vi "html_read.vi"() -> ()   [LabVIEW 2015]
uses:
  <vilib>/httpClient/LabVIEWHTTPClient.lvlib
panel:
  out "body 2":string
  in  "File Type":string=".CSV"
  in  "File Prefix":string="GPSLOG"
  out "Number of Files":i32
  out "body":string
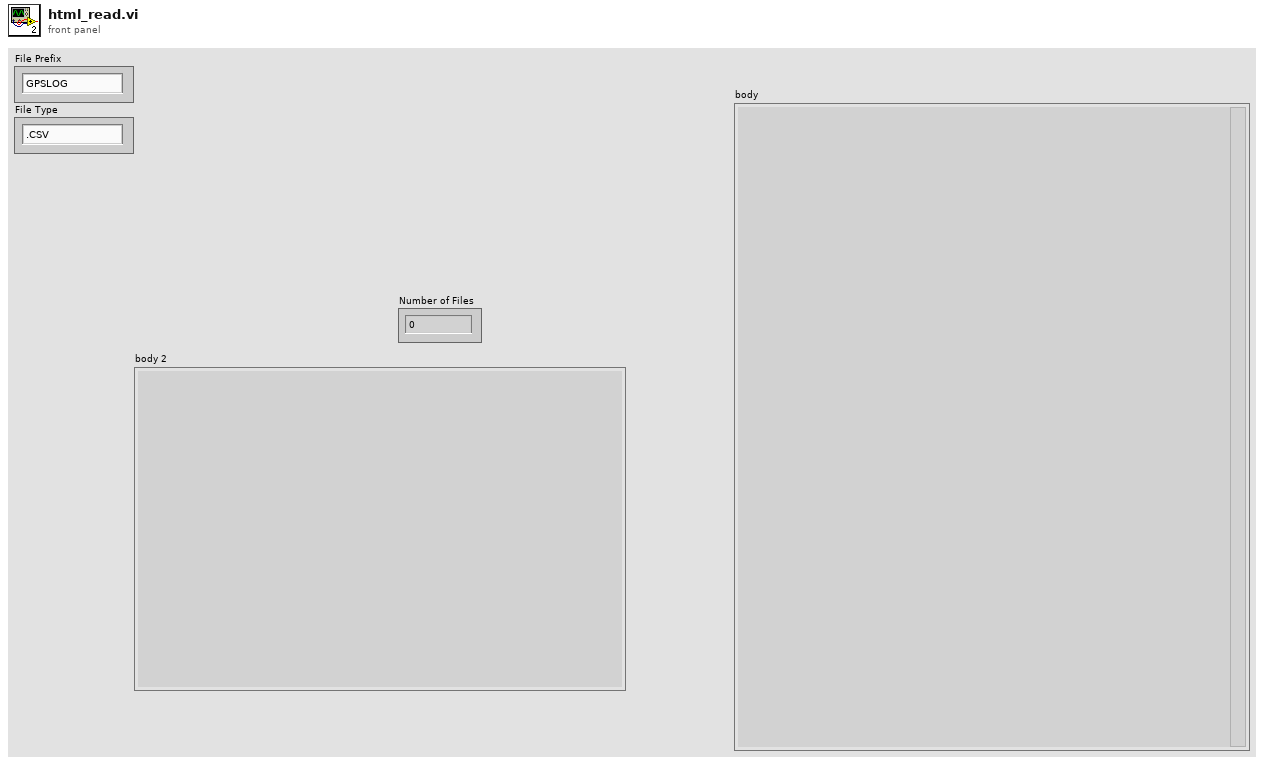
[diagram p1: front panel]
types:
  T1 = typedef "LabVIEWHTTPClient.lvlib/ClientHandle.ctl" = refnum<k1>
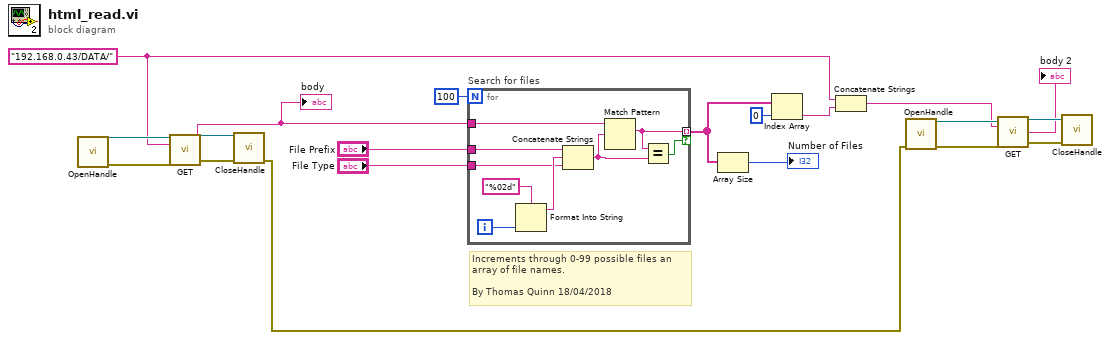
[diagram p0: block diagram]
diagram:
  w4 = "192.168.0.43/DATA/" ("url")
  # "Increments through 0-99 possible files an array of file names.\n\nBy Thomas Quinn 18/04/2018"
  n1 = call <vilib>:"OpenHandle.vi"() -> ("client handle out"=w20:T1, "error out"=w19:errorcluster)  [unwired: 14 in]
  n2 = call <vilib>:"GET.vi"("client handle"=w20, "url"=w4, "error in (no error)"=w19) -> ("client handle out"=w13:T1, "body"=w17:string, "error out"=w12:errorcluster)  [unwired: 9 in, 1 out]
  "body" <- w17
  n3 = call <vilib>:"CloseHandle.vi"("client handle"=w13, "error in (no error)"=w12) -> ("error out"=w9:errorcluster)  [unwired: 13 in]
  n4 = for "Search for files" {
    N: 100 -> [_]
    tunnel: "File Prefix" -> [w26]
    tunnel: w17 -> [w29]
    tunnel: [w21] -> w6 mode=indexing if=w22
    tunnel: "File Type" -> [w24]
    i -> [w28]
    n5 = Format Into String(format string="%02d", w28) -> (resulting string=w25:string)  [unwired: 2 in, 1 out]
    n6 = Concatenate Strings(w26, w25, w24) -> (w23:string)
    n7 = Match Pattern(string=w29, regular expression=w23) -> (match substring=w21:string)  [unwired: 1 in, 3 out]
    n8 = Equal?(x=w21, y=w23) -> (x = y?=w22:bool)
  }
  n9 = Array Size(array=w6) -> (size(s)=→"Number of Files":i32)
  n10 = Index Array(array=w6, index=0) -> (element=w3:string)
  n11 = Concatenate Strings(w4, w3) -> (w2:string)
  n12 = call <vilib>:"OpenHandle.vi"("error in (no error)"=w9) -> ("client handle out"=w8:T1, "error out"=w10:errorcluster)  [unwired: 13 in]
  n13 = call <vilib>:"GET.vi"("client handle"=w8, "url"=w2, "error in (no error)"=w10) -> ("client handle out"=w7:T1, "body"=→"body 2":string, "error out"=w11:errorcluster)  [unwired: 9 in, 1 out]
  n14 = call <vilib>:"CloseHandle.vi"("client handle"=w7, "error in (no error)"=w11) -> ()  [unwired: 13 in, 1 out]
